vi "OLS_LevelZeroVerification.vi"() -> ()   [LabVIEW 2024]
doc: "Used to verify and calculate the Level Zero offset value. The User is Prompted for their NAME, then the Level is set to 5 evaluation Set Points (SP). Onece the SP is reached the User should measure the oil level from the datum then recored the MEASURED Level in Inches when prompted. Once all five measuremnts are complete, the results are fit using LSR, a residual plot is displayed and the user is prompted to select an Excel workbook to which the results are appended on sheet 1. \n\nUse the STOP button to interrupt and end the Zero process."
uses:
  Control Definitions/Def_CalState_Enum.ctl
  Control Definitions/Def_PumpSpeed.ctl
  Control Definitions/DEF_PumpManCtl.ctl
  Control Definitions/DEF_PumpParams.ctl
  <vilib>/Analysis/NI_AALPro.lvlib
panel:
  out "Constant":dbl format="%.4g"
  out "Auto/!Man":bool=TRUE
  in  "Pump Params":T1={"Empty Inches"=1.1, "Full Inches"=7.2, "RNG_SLOW"=0.5, "RNG_CREEP"=0.007, "RNG_STOP "=0.002, "VISA resource name"="COM4", "SPD_SLOW"=30, "SPD_CREEP"=10, "SPD_FAST"=100, "Zero template"=path "C:/AllenProjects/PWC-OLS/$Calibrtation/CAL_Level_RnR_241105.xlsx", "zero  Settle sec"=5.0} {"RNG_STOP" format="%#_13g"; "RNG_CREEP" format="%#_13g"; "RNG_SLOW" format="%#_13g"}
  in  "Pump Manual Controls":T2={"Pump Speed"=enum."STOP", "FILL"=FALSE, "Drain"=FALSE, "Auto/!Man"=TRUE}
  out "Msg":string
  out "Pump Status":bool=TRUE
  in  "Sim Level":bool
  out "Residual Plot":dbl[](graph)=[-0.0, -0.0, -0.0, -0.0, -0.0]
  out "Offest":dbl=-0.0 format="%.4g"
  out "Slope":dbl=-0.0 format="%.4g"
  out "Time":string="11/17/2024 3:56 PM"
  out "Name":string="rob"
  in  "Stop Pump":bool=TRUE
  out "Calibration":cluster{"SP":dbl, "Laser":dbl, "Measure":dbl}[](array[cluster])=[{"SP"=1.1, "Laser"=1.102, "Measure"=0.0}, {"SP"=2.7229265223579855, "Laser"=2.7239999999999855, "Measure"=0.0}, {"SP"=4.174679755518124, "Laser"=4.173999999999982, "Measure"=0.0}, {"SP"=5.682906773962424, "Laser"=5.6819999999999755, "Measure"=0.0}, {"SP"=7.199999999999999, "Laser"=7.203999999999969, "Measure"=0.0}] {"Measure" format="%.3g"; "Laser" format="%.3g"; "SP" format="%.3g"}
  out "Count":i32=5
  out "Pump Speed Out":T3=enum."CREEP"
  out "State Var":T4=enum."Done"
  in  "stop":bool
  out "Level PV":dbl(slide)=7.203999999999969 scale=0.0..10.0
  in  "Level SP":dbl(slide)=7.199999999999999 scale=0.0..10.0
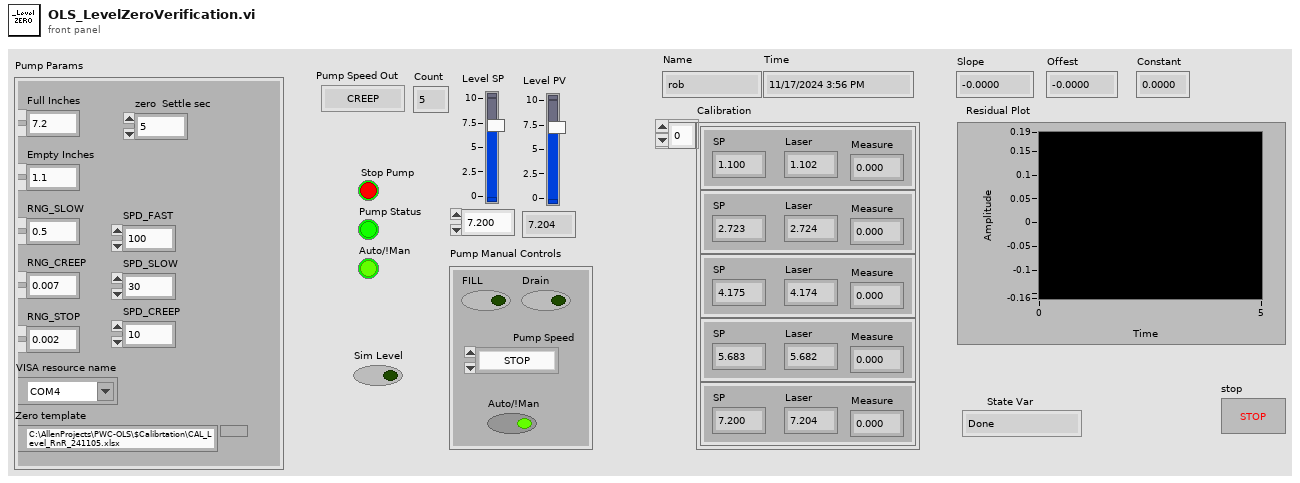
[diagram p1: front panel]
types:
  T1 = typedef "DEF_PumpParams.ctl" = cluster{"Empty Inches":dbl, "Full Inches":dbl, "RNG_SLOW":dbl, "RNG_CREEP":dbl, "RNG_STOP ":dbl, "VISA resource name":refnum<visa-resource-name>, "SPD_SLOW":i32, "SPD_CREEP":i32, "SPD_FAST":i32, "Zero template":path, "zero  Settle sec":dbl}
  T2 = typedef "DEF_PumpManCtl.ctl" = cluster{"Pump Speed":T3, "FILL":bool, "Drain":bool, "Auto/!Man":bool}
  T3 = typedef "Def_PumpSpeed.ctl" = enum16{"FAST", "SLOW", "CREEP", "STOP"}
  T4 = typedef "Def_CalState_Enum.ctl" = enum16{"Start", "Get Info", "Get SP", "Going to SP", "Wait Settle", "Get Measure", "Save Measure", "Done", "Manual"}
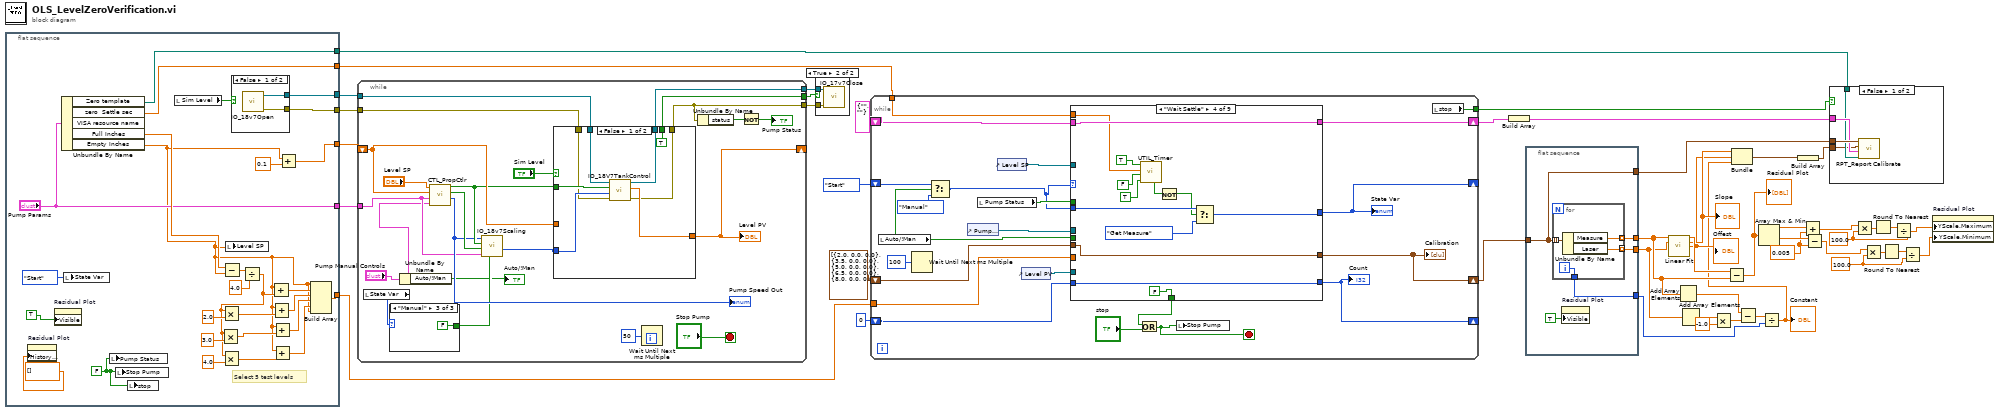
[diagram p0: block diagram]
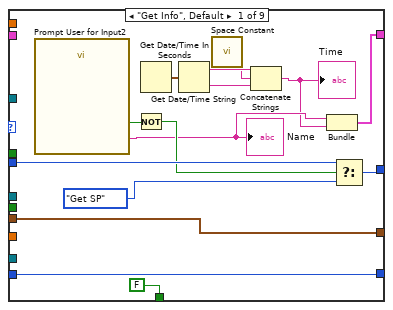
[diagram p5: hidden frame]
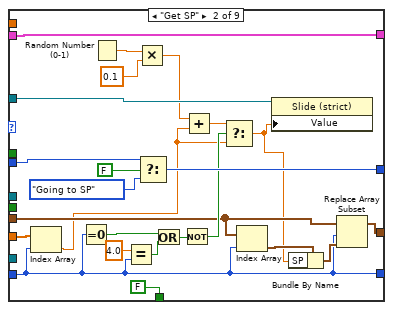
[diagram p6: hidden frame]
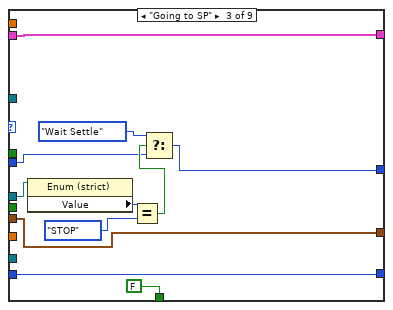
[diagram p7: hidden frame]
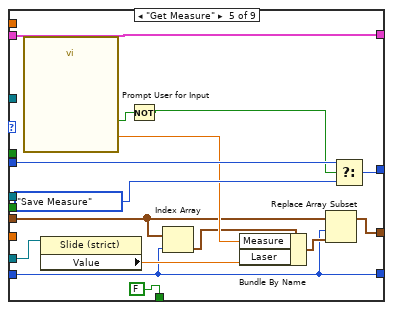
[diagram p8: hidden frame]
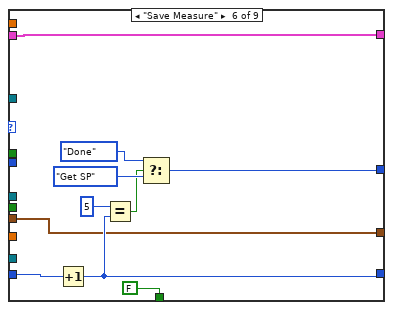
[diagram p9: hidden frame]
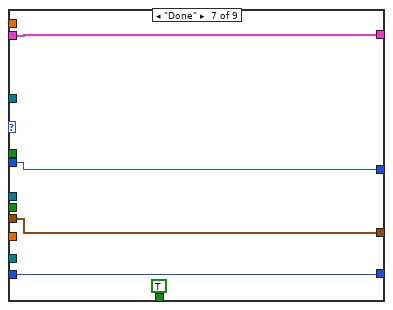
[diagram p10: hidden frame]
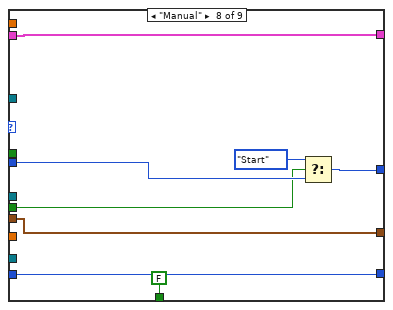
[diagram p11: hidden frame]
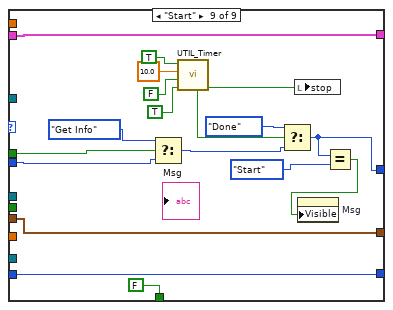
[diagram p12: hidden frame]
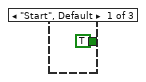
[diagram p13: hidden frame]
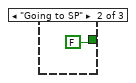
[diagram p14: hidden frame]
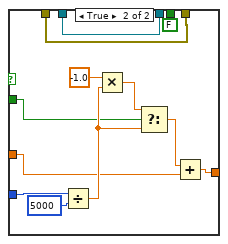
[diagram p15: hidden frame]
diagram:
  w18 = 100.0 ("y")
  w25 = 100.0 ("y")
  w41 = 0.005 ("y")
  n1 = flat-sequence {
    tunnel: [w50] -> w47
    tunnel: [w61] -> w33
    tunnel: [w59] -> w30
    tunnel: [w58] -> w29
    tunnel: ["Pump Params"] -> w17
    tunnel: [w49] -> w13
    tunnel: [w48] -> w12
    frame #0 {
      w57 = FALSE
      # "Select 5 test levels"
      n2 = property on="Residual Plot" class="WFChart (strict)"("History Data"=dbl[] []) -> ()  [unwired: 2 in, 2 out]
      n3 = property on="Residual Plot" class="WFChart (strict)"("Visible"=TRUE) -> ()  [unwired: 2 in, 2 out]
      n4 = Unbundle By Name("Pump Params") -> ("Zero template"=w49:path, "zero  Settle sec"=w48:dbl, "Full Inches"=w56:dbl, "Empty Inches"=w51:dbl)  [unwired: 1 out]
      n5 = local write "State Var"(Def_CalState_Enum."Start" ("State Var")) -> ()
      n6 = local write "Pump Status"(w57) -> ()
      n7 = local write "Stop Pump"(w57) -> ()
      n8 = local write "stop"(w57) -> ()
      n9 = local read "Sim Level"() -> (w53:bool)
      n10 = Subtract(x=w56, y=w51) -> (x-y=w73:dbl)
      n11 = local write "Level SP"(w51) -> ()
      n12 = case shown="False" w53 {
        tunnel: [w77 _] -> w59
        tunnel: [w76 _] -> w58
        frame False {
          n13 = call "IO_18v7Open.vi"() -> ("error out"=w76:errorcluster, "VISA Refnum out"=w77:refnum<visa-resource-name>)  [unwired: 10 in]
        }
        frame True {
        }
      }
      n14 = Divide(x=w73, y=4.0) -> (x/y=w60:dbl)
      n15 = Multiply(x=w60, y=3.0) -> (x*y=w66:dbl)
      n16 = Multiply(x=w60, y=2.0) -> (x*y=w69:dbl)
      n17 = Multiply(x=w60, y=4.0) -> (x*y=w65:dbl)
      n18 = Add(x=w51, y=w60) -> (x+y=w70:dbl)
      n19 = Add(x=w51, y=w69) -> (x+y=w64:dbl)
      n20 = Add(x=w51, y=w66) -> (x+y=w63:dbl)
      n21 = Add(x=w51, y=w65) -> (x+y=w62:dbl)
      n22 = Add(x=w51, y=0.1) -> (x+y=w50:dbl)
      n23 = Build Array(w51, w70, w64, w63, w62, w51) -> (w61:dbl[])
    }
  }
  n24 = while {
    shift-right: [w95] -> _
    shift-left: w47 -> [w97]
    tunnel: [w93] -> w32
    tunnel: [w86] -> w31
    tunnel: w30 -> [w92]
    tunnel: w29 -> [w91]
    tunnel: w17 -> [w83]
    tunnel: [w80] -> w16
    stop <- "Stop Pump" stop-if-true
    n25 = local read "State Var"() -> (w82:T4)
    n26 = case shown="\"Manual\"" w82 {
      tunnel: [TRUE FALSE FALSE] -> w81
      frame "Start", Default {
      }
      frame "Going to SP" {
      }
      frame "Manual" {
      }
    }
    n27 = Unbundle By Name("Pump Manual Controls") -> ("Auto/!Man"=→"Auto/!Man":bool)
    n28 = call "CTL_PropCtlr.vi"("Pump Manual Controls"="Pump Manual Controls", "Pump Params"=w83, "Level PV"=w97, "Level SP"="Level SP") -> ("Pump Speed Out"=w88:T3, "X< Neg"=w90:bool, "X>Pos"=w89:bool)  [unwired: 4 in, 1 out]
    "Pump Speed Out" <- w88
    n29 = call "IO_18v7Scaling.vi"("!Enabled"=w81, "Pump Params"=w83, "Drain"=w90, "Fill"=w89, "Pump Speed"=w88) -> ("Speed Out"=w87:i32)  [unwired: 5 in, 1 out]
    n30 = case shown="False" "Sim Level" {
      tunnel: w97 -> [_ w113]
      tunnel: [w110 w121] -> w95
      tunnel: w89 -> [w109 w111]
      tunnel: w87 -> [w108 w115]
      tunnel: [w107 w117] -> w93
      tunnel: [w106 w116] -> w86
      tunnel: w92 -> [w105 w117]
      tunnel: w91 -> [w104 w116]
      tunnel: [TRUE FALSE] -> w80
      frame False {
        n31 = call "IO_18V7TankControl.vi"("error in"=w104, "Speed"=w108, "Fill!Drain"=w109, "VISA Refnum in"=w105) -> ("error out"=w106:errorcluster, "Laser Raw"=w110:sgl, "VISA Refnum out"=w107:refnum<visa-resource-name>)  [unwired: 4 in, 1 out]
      }
      frame True {
        n32 = Divide(x=w115, y=5000) -> (x/y=w119:dbl)
        n33 = Multiply(x=-1.0 ("y"), y=w119) -> (x*y=w120:dbl)
        n34 = Select(t=w120, s=w111, f=w119) -> (s? t:f=w114:dbl)
        n35 = Add(x=w114, y=w113) -> (x+y=w121:dbl)
      }
    }
    "Level PV" <- w95
    n36 = Wait Until Next ms Multiple(millisecond multiple=u32 50) -> ()  [unwired: 1 out]
    n37 = Unbundle By Name(w86) -> ("status"=w85:bool)
    n38 = Not(x=w85) -> (.not. x?=→"Pump Status":bool)
  }
  n39 = case shown="True" w16 {
    tunnel: w32 -> [_ w124]
    tunnel: w31 -> [_ w123]
    frame False {
    }
    frame True {
      n40 = call "IO_17v7Close.vi"("error in (no error)"=w123, "VISA Refnum in"=w124) -> ()  [unwired: 10 in]
    }
  }
  n41 = while {
    shift-right: [w145] -> _
    shift-left: Def_CalState_Enum."Start" ("f") -> [w129]
    shift-right: [w138] -> _
    shift-left: 0 -> [w141]
    shift-right: [w136] -> w14
    shift-left: cluster{"SP":dbl, "Laser":dbl, "Measure":dbl}[] [{"SP"=2.0, "Laser"=0.0, "Measure"=0.0}, {"SP"=3.5, "Laser"=0.0, "Measure"=0.0}, {"SP"=5.0, "Laser"=0.0, "Measure"=0.0}, {"SP"=6.5, "Laser"=0.0, "Measure"=0.0}, {"SP"=8.0, "Laser"=0.0, "Measure"=0.0}] ("Calibration") -> [w137]
    shift-right: [w135] -> w36
    shift-left: cluster{"Name":string, string} {"Name"="", ""} -> [w134]
    tunnel: w33 -> [w133]
    tunnel: [w131] -> w28
    tunnel: w12 -> [w125]
    stop <- w140 stop-if-true
    n42 = local read "Auto/!Man"() -> (w126:bool)
    n43 = Wait Until Next ms Multiple(millisecond multiple=u32 100) -> ()  [unwired: 1 out]
    n44 = Select(t=w129, s=w126, f=Def_CalState_Enum."Manual") -> (s? t:f=w128:T4)
    n45 = control-ref of="Pump Speed Out"() -> (w144:refnum<vi>)
    n46 = local read "Pump Status"() -> (w130:bool)
    n47 = control-ref of="Level SP"() -> (w142:refnum<vi>)
    n48 = control-ref of="Level PV"() -> (w139:refnum<vi>)
    n49 = case shown="\"Wait Settle\"" w128 {
      tunnel: [w159 w183 w196 w198 w224 w227 w239 w244 w250] -> w145
      tunnel: w128 -> [w160 w184 w192 w208 w223 _ w239 w243 w262]
      tunnel: w144 -> [_ _ w191 _ _ _ _ _ _]
      tunnel: w141 -> [w158 w163 w189 w207 w211 w234 w238 w245 w264]
      tunnel: [w158 w163 w189 w207 w211 w233 w238 w245 w264] -> w138
      tunnel: [FALSE FALSE FALSE FALSE FALSE FALSE TRUE FALSE FALSE] -> w143
      tunnel: w142 -> [_ w181 _ _ _ _ _ _ _]
      tunnel: w139 -> [_ _ _ _ w215 _ _ _ _]
      tunnel: w137 -> [w156 w167 w187 w200 w212 w226 w236 w246 w265]
      tunnel: [w156 w166 w187 w200 w216 w226 w236 w246 w265] -> w136
      tunnel: [w149 w179 w186 w199 w213 w225 w235 w247 w263] -> w135
      tunnel: w134 -> [_ w179 w186 w199 w213 w225 w235 w247 w263]
      tunnel: w133 -> [_ w169 _ _ _ _ _ _ _]
      tunnel: w130 -> [_ _ _ _ _ _ _ _ w261]
      tunnel: w126 -> [_ _ _ _ _ _ _ w241 _]
      tunnel: w125 -> [_ _ _ w197 _ _ _ _ _]
      frame "Get Info", Default {
        n50 = call "Prompt User for Input2"() -> ("Name"=w151:string, "OK"=w155:bool)  [unwired: 17 in, 1 out]
        "Name" <- w151
        n51 = Not(x=w155) -> (.not. x?=w154:bool)
        n52 = Get Date/Time In Seconds() -> (seconds since 1Jan1904=w153:timestamp)
        n53 = Get Date/Time String(seconds (now)=w153) -> (date string=w152:string, time string=w148:string)  [unwired: 2 in]
        n54 = call <vilib>:"Space Constant.vi"() -> ("String"=w147:string)
        n55 = Concatenate Strings(w152, w147, w148) -> (w150:string)
        "Time" <- w150
        n56 = Bundle("Name"=w151, w150) -> (w149:cluster{"Name":string, string})  [unwired: 1 in]
        n57 = Select(t=w160, s=w154, f=Def_CalState_Enum."Get SP") -> (s? t:f=w159:T4)
      }
      frame "Get SP" {
        n58 = Index Array(array=w169, index=w163) -> (element=w165:dbl)
        n59 = Equal To 0?(x=w163) -> (x = 0?=w173:bool)
        n60 = Random Number (0-1)() -> (number: 0 to 1=w177:dbl)
        n61 = Equal?(x=4.0 ("y"), y=w163) -> (x = y?=w174:bool)
        n62 = Multiply(x=w177, y=0.1) -> (x*y=w176:dbl)
        n63 = Select(t=w184, s=FALSE ("s 2"), f=Def_CalState_Enum."Going to SP") -> (s? t:f=w183:T4)
        n64 = Or(x=w173, y=w174) -> (x .or. y?=w172:bool)
        n65 = Not(x=w172) -> (.not. x?=w171:bool)
        n66 = Add(x=w176, y=w165) -> (x+y=w170:dbl)
        n67 = Select(t=w170, s=w171, f=w165) -> (s? t:f=w162:dbl)
        n68 = Index Array(array=w167, index=w163) -> (element=w168:cluster{"SP":dbl, "Laser":dbl, "Measure":dbl})
        n69 = property class="Slide (strict)"(reference=w181, "Value"=w162) -> ()  [unwired: 1 in, 2 out]
        n70 = Bundle By Name(cluster=w168, "SP"=w162) -> (w164:cluster{"SP":dbl, "Laser":dbl, "Measure":dbl})
        n71 = Replace Array Subset(array=w167, new element=w164, index=w163) -> (w166:cluster{"SP":dbl, "Laser":dbl, "Measure":dbl}[])
      }
      frame "Going to SP" {
        n72 = property class="Enum (strict)"(reference=w191) -> ("Value"=w190:T3)  [unwired: 1 in, 2 out]
        n73 = Equal?(x=w190, y=Def_PumpSpeed."STOP") -> (x = y?=w195:bool)
        n74 = Select(t=Def_CalState_Enum."Wait Settle" ("f"), s=w195, f=w192) -> (s? t:f=w196:T4)
      }
      frame "Wait Settle" {
        n75 = call "UTIL_Timer.vi"("Auto Reset"=TRUE, "Reset"=FALSE, "Time (sec)"=w197, "Start"=TRUE) -> ("TO Trig"=w203:bool)  [unwired: 2 in, 5 out]
        n76 = Not(x=w203) -> (.not. x?=w202:bool)
        n77 = Select(t=w208, s=w202, f=Def_CalState_Enum."Get Measure") -> (s? t:f=w198:T4)
      }
      frame "Get Measure" {
        n78 = call "Prompt User for Input"() -> ("Measure"=w220:dbl, "OK"=w219:bool)  [unwired: 17 in, 1 out]
        n79 = property class="Slide (strict)"(reference=w215) -> ("Value"=w214:dbl)  [unwired: 1 in, 2 out]
        n80 = Not(x=w219) -> (.not. x?=w218:bool)
        n81 = Index Array(array=w212, index=w211) -> (element=w210:cluster{"SP":dbl, "Laser":dbl, "Measure":dbl})
        n82 = Bundle By Name(cluster=w210, "Measure"=w220, "Laser"=w214) -> (w217:cluster{"SP":dbl, "Laser":dbl, "Measure":dbl})
        n83 = Replace Array Subset(array=w212, new element=w217, index=w211) -> (w216:cluster{"SP":dbl, "Laser":dbl, "Measure":dbl}[])
        n84 = Select(t=w223, s=w218, f=Def_CalState_Enum."Save Measure") -> (s? t:f=w224:T4)
      }
      frame "Save Measure" {
        n85 = Increment(x=w234) -> (x+1=w233:i32)
        n86 = Equal?(x=5, y=w233) -> (x = y?=w229:bool)
        n87 = Select(t=Def_CalState_Enum."Done" ("f"), s=w229, f=Def_CalState_Enum."Get SP") -> (s? t:f=w227:T4)
      }
      frame "Done" {
      }
      frame "Manual" {
        n88 = Select(t=Def_CalState_Enum."Start", s=w241, f=w243) -> (s? t:f=w244:T4)
      }
      frame "Start" {
        n89 = Select(t=Def_CalState_Enum."Get Info", s=w261, f=w262) -> (s? t:f=w253:T4)
        n90 = call "UTIL_Timer.vi"("Auto Reset"=TRUE, "Reset"=FALSE, "Time (sec)"=10.0, "Start"=TRUE) -> ("Timed Out"=w251:bool, "TO Trig"=w252:bool)  [unwired: 2 in, 4 out]
        n91 = Select(t=Def_CalState_Enum."Done", s=w252, f=w253) -> (s? t:f=w250:T4)
        n92 = local write "stop"(w251) -> ()
        n93 = Equal?(x=w250, y=Def_CalState_Enum."Start" ("t")) -> (x = y?=w248:bool)
        n94 = property on="Msg" class="Str"("Visible"=w248) -> ()  [unwired: 2 in, 2 out]
      }
    }
    "State Var" <- w145
    "Count" <- w138
    "Calibration" <- w136
    n95 = Or(x=w143, y="stop") -> (x .or. y?=w140:bool)
    n96 = local write "Stop Pump"(w140) -> ()
    n97 = local read "stop"() -> (w131:bool)
  }
  n98 = Build Array(w36) -> (w35:cluster{"Name":string, string}[])
  n99 = flat-sequence {
    tunnel: [w270] -> w11
    tunnel: [w269] -> w10
    tunnel: w14 -> [w267]
    tunnel: [w267] -> w15
    tunnel: [w266] -> w4
    frame #0 {
      n100 = for {
        tunnel: w267 -> [w274] mode=indexing
        tunnel: [w273] -> w270 mode=indexing
        tunnel: [w272] -> w269 mode=indexing
        tunnel: [w271] -> w266
        i -> [w271]
        n101 = Unbundle By Name(w274) -> ("Measure"=w273:dbl, "Laser"=w272:dbl)
      }
      n102 = property on="Residual Plot" class="WFChart (strict)"("Visible"=TRUE) -> ()  [unwired: 2 in, 2 out]
    }
  }
  n103 = call <vilib>:"Linear Fit.vi"("Y"=w11, "X"=w10) -> ("Best Linear Fit"=w44:dbl[], "slope"=w39:dbl, "intercept"=w38:dbl)  [unwired: 9 in, 2 out]
  "Slope" <- w39
  "Offest" <- w38
  n104 = Add Array Elements(numeric array=w11) -> (sum=w6:dbl)
  n105 = Add Array Elements(numeric array=w10) -> (sum=w9:dbl)
  n106 = Multiply(x=w9, y=-1.0) -> (x*y=w7:dbl)
  n107 = Subtract(x=w44, y=w11) -> (x-y=w43:dbl[])
  "Residual Plot" <- w43
  n108 = Subtract(x=w6, y=w7) -> (x-y=w5:dbl)
  n109 = Array Max & Min(array=w43) -> (max value=w40:dbl, min value=w42:dbl)  [unwired: 2 out]
  n110 = Divide(x=w5, y=w4) -> (x/y=w3:dbl)
  "Constant" <- w3
  n111 = Bundle("slope"=w39, "intercept"=w38, w3) -> (w2:cluster{"slope":dbl, "intercept":dbl, dbl})  [unwired: 1 in]
  n112 = Build Array(w2) -> (w1:cluster{"slope":dbl, "intercept":dbl, dbl}[])
  n113 = Add(x=w40, y=w41) -> (x+y=w24:dbl)
  n114 = Subtract(x=w42, y=w41) -> (x-y=w19:dbl)
  n115 = case shown="False" w28 {
    tunnel: w15 -> [w278 _]
    tunnel: w35 -> [w277 _]
    tunnel: w13 -> [w276 _]
    tunnel: w1 -> [w275 _]
    frame False {
      n116 = call "RPT_Report Calibrate.vi"("template"=w276, "Info"=w277, "LinEq"=w275, "Calibration"=w278) -> ()  [unwired: 8 in]
    }
    frame True {
    }
  }
  n117 = Multiply(x=w24, y=w25) -> (x*y=w26:dbl)
  n118 = Multiply(x=w19, y=w18) -> (x*y=w21:dbl)
  n119 = Round To Nearest(number=w26) -> (nearest integer value=w27:dbl)
  n120 = Round To Nearest(number=w21) -> (nearest integer value=w22:dbl)
  n121 = Divide(x=w27, y=w25) -> (x/y=w23:dbl)
  n122 = Divide(x=w22, y=w18) -> (x/y=w20:dbl)
  n123 = property on="Residual Plot" class="WFChart (strict)"("YScale.Maximum"=w23, "YScale.Minimum"=w20) -> ()  [unwired: 2 in, 2 out]
